vi "Servo.vi"() -> ()   [LabVIEW 2013]
uses:
  <vilib>/rvi/Emulation/niFpgaSctlEmulationGetInTimedLoop.vi
  <vilib>/rvi/Emulation/niFpgaEmulationReportErrorSimple.vi
  <vilib>/rvi/Emulation/niFpgaGetClockAttributes.vi
  <vilib>/rvi/eio/common/nirviEmuTemplateMethod_errors.vi
  <vilib>/rvi/Emulation/niFpgaCriticalErrorInLSC.vi
  <vilib>/eio/EIONode/EIONode.xnode
panel:
  in  "servo 6":u32=1500
  in  "Count(uSec)":u32=5000
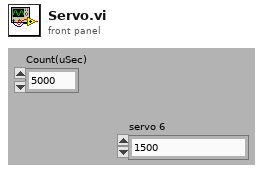
[diagram p1: front panel]
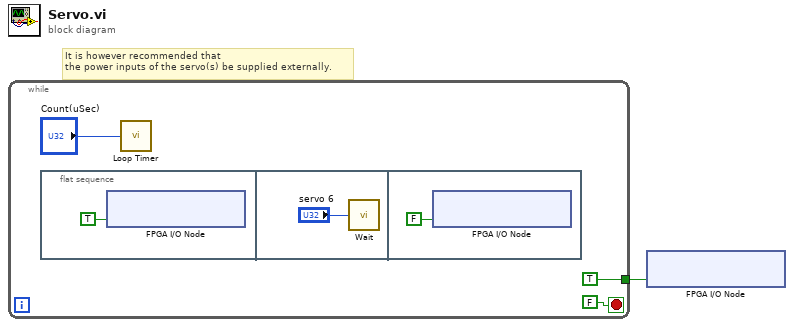
[diagram p0: block diagram]
diagram:
  # "It is however recommended that\nthe power inputs of the servo(s) be supplied externally."
  n1 = while {
    tunnel: [TRUE] -> w1
    stop <- FALSE stop-if-true
    n2 = flat-sequence {
      frame #0 {
        n3 = xnode "FPGA I/O Node"("ConnectorA/DIO0"=TRUE) -> ()  [unwired: 1 in, 1 out]
      }
      frame #1 {
        n4 = call "Wait"("Count(uSec)"="servo 6") -> ()  [unwired: 1 out]
      }
      frame #2 {
        n5 = xnode "FPGA I/O Node"("ConnectorA/DIO0"=FALSE) -> ()  [unwired: 1 in, 1 out]
      }
    }
    n6 = call "Loop Timer"("Count(uSec)"="Count(uSec)") -> ()  [unwired: 1 out]
  }
  n7 = xnode "FPGA I/O Node"("ConnectorA/DIO0"=w1) -> ()  [unwired: 1 in, 1 out]
